vi "Sine_wave Init 1d LUT (2).vi"() -> (3 "Init Data Out":u16[](array[numeric]))   [LabVIEW 2018]
uses:
  <vilib>/measure/NI_MABase.lvlib
panel:
  in  "DC offset":dbl
  in  "meas. time":dbl
  in  "dt FPGA":dbl
  in  "sampling info":cluster{"Fs":dbl, "#s":dbl}={"Fs"=1000.0, "#s"=1000.0} {"Fs" format="%.2p"}
  in  "amplitude\n[V]":dbl
  in  "Frequency \n[1/s]":dbl
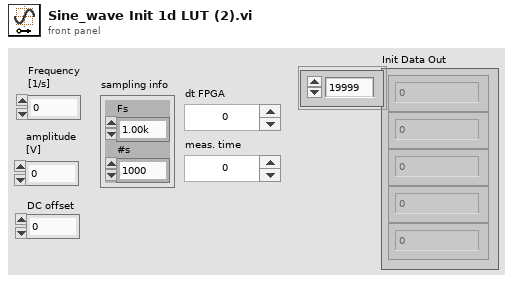
[diagram p1: front panel]
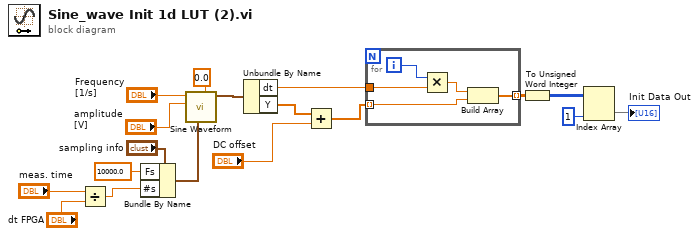
[diagram p0: block diagram]
diagram:
  n1 = Divide(x="meas. time", y="dt FPGA") -> (x/y=w10:dbl)
  n2 = Bundle By Name(cluster="sampling info", "Fs"=10000.0, "#s"=w10) -> (w8:cluster{"Fs":dbl, "#s":dbl})
  n3 = call <vilib>:"Sine Waveform.vi"("offset"=0.0, "sampling info"=w8, "amplitude"="amplitude\n[V]", "frequency"="Frequency \n[1/s]") -> ("signal out"=w18:waveform(dbl))  [unwired: 6 in, 1 out]
  n4 = Unbundle By Name(w18) -> ("dt"=w14:dbl, "Y"=w5:dbl[])
  n5 = Add(x=w5, y="DC offset") -> (x+y=w4:dbl[])
  n6 = for {
    tunnel: w4 -> [w23] mode=indexing
    tunnel: w14 -> [w21]
    tunnel: [w19] -> w3 mode=indexing
    i -> [w22]
    n7 = Multiply(x=w22, y=w21) -> (x*y=w20:dbl)
    n8 = Build Array(w20, w23) -> (w19:dbl[])
  }
  n9 = To Unsigned Word Integer(number=w3) -> (unsigned 16bit integer=w2:u16[][])
  n10 = Index Array(array=w2, index (col)=1 ("disabled index (col)")) -> (element=→"Init Data Out":u16[])  [unwired: 1 in]
